vi "load_automatic.vi"(8 "error in (no error)":errorcluster) -> (0 "error out":errorcluster, 2 "replaced_step(s)":bool, 3 "automatic_steps out":variant)   [LabVIEW 2015, in "example_02.lvlib"]
doc: "load_automatic.vi will add automatic steps as variant attributes to an empty variant."
uses:
  example_02.lvlib
  <userlib>/antonio-alexander/lv-recipe-machine/public/_controls/step.ctl
  <userlib>/antonio-alexander/lv-recipe-machine/public/_controls/vi_reference_type.ctl
  _controls/steps_actions.ctl
  <userlib>/antonio-alexander/lv-recipe-machine/public/_controls/vi_reference_automatic_step.ctl
  <userlib>/antonio-alexander/lv-recipe-machine/public/_controls/vi_reference_criteria.ctl
  <userlib>/antonio-alexander/lv-recipe-machine/public/_controls/vi_reference_launch.ctl
  <userlib>/antonio-alexander/lv-recipe-machine/public/_controls/vi_reference_manual_action.ctl
  <userlib>/antonio-alexander/lv-recipe-machine/public/_controls/vi_reference_transition.ctl
  automatic_steps/transition.vi
  automatic_steps/automatic_step_address.vi
  automatic_steps/automatic_step_city.vi
  automatic_steps/automatic_step_state.vi
  automatic_steps/automatic_step_submit.vi
  automatic_steps/automatic_step_finish.vi
  <userlib>/antonio-alexander/lv-recipe-machine/lv-recipe-machine.lvlib
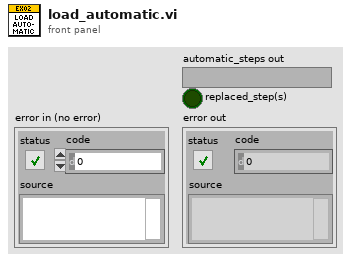
[diagram p1: front panel]
types:
  T1 = typedef "lv-recipe-machine.lvlib/vi_reference_type.ctl" = enum16{"<vi_reference_type>", "manual_action", "auto_step", "auto_criteria", "auto_transition", "auto_launcher", "<null>"}
  T2 = typedef "lv-recipe-machine.lvlib/vi_reference_transition.ctl" = refnum<vi>
  T3 = typedef "lv-recipe-machine.lvlib/vi_reference_manual_action.ctl" = refnum<vi>
  T4 = typedef "lv-recipe-machine.lvlib/vi_reference_launch.ctl" = refnum<vi>
  T5 = typedef "lv-recipe-machine.lvlib/vi_reference_criteria.ctl" = refnum<vi>
  T6 = typedef "lv-recipe-machine.lvlib/vi_reference_automatic_step.ctl" = refnum<vi>
  T7 = typedef "example_02.lvlib/steps_actions.ctl" = enum16{"<steps_actions>", "auto_start", "auto_first_name", "auto_last_name", "auto_address", "auto_city", "auto_state", "auto_zip_code", "auto_submit", "auto_finish", "transition", "<null>"}
  T8 = typedef "lv-recipe-machine.lvlib/step.ctl" = cluster{"name":string, "vi_reference":variant}
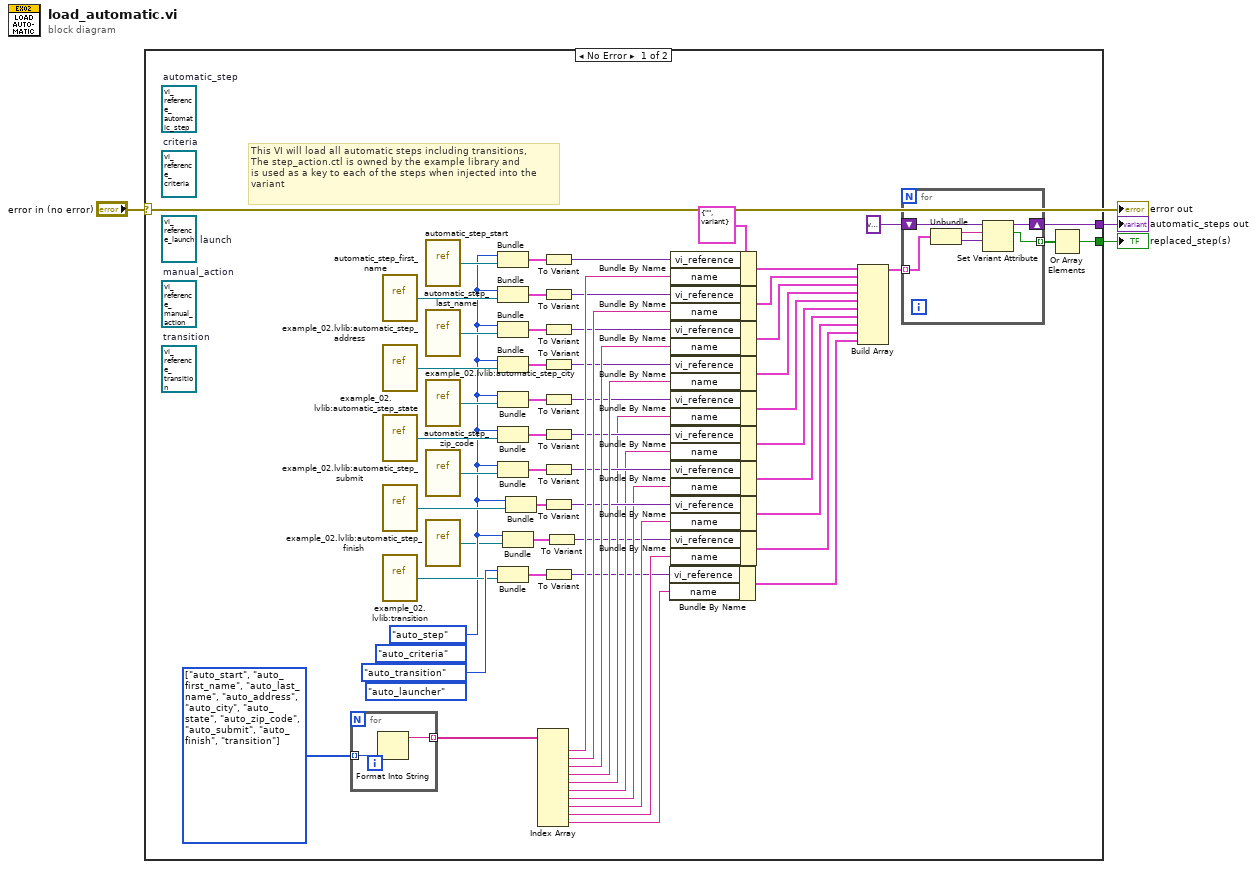
[diagram p0: block diagram]
diagram:
  n1 = case shown="No Error" "error in (no error)" {
    tunnel: [w63 _] -> w3
    tunnel: [w60 _] -> w2
    frame No Error {
      (unwired) T2 refnum  # transition
      (unwired) T3 refnum  # manual_action
      (unwired) T4 refnum  # launch
      (unwired) T5 refnum  # criteria
      (unwired) T6 refnum  # automatic_step
      (unwired) vi_reference_type."auto_launcher" ("vi_reference_type")
      w55 = T7[] [enum."auto_start", enum."auto_first_name", enum."auto_last_name", enum."auto_address", enum."auto_city", enum."auto_state", enum."auto_zip_code", enum."auto_submit", enum."auto_finish", enum."transition"] items=["<steps_actions>", "auto_start", "auto_first_name", "auto_last_name", "auto_address", "auto_city", "auto_state", "auto_zip_code", "auto_submit", "auto_finish", "transition", "<null>"]
      (unwired) vi_reference_type."auto_criteria" ("vi_reference_type")
      w8 = vi_reference_type."auto_step" ("vi_reference_type")
      w11 = T8 {"name"="", "vi_reference"=variant(refnum<vi> refnum)} ("step")
      # "This VI will load all automatic steps including transitions, \nThe step_action.ctl is owned by the example library and\nis used as a key to each of the steps when injected into the\nvariant"
      n2 = for {
        tunnel: w55 -> [w65] mode=indexing
        tunnel: [w64] -> w54 mode=indexing
        n3 = Format Into String(w65) -> (resulting string=w64:string)  [unwired: 3 in, 1 out]
      }
      n4 = vi-ref "automatic_step_first_name.vi"() -> (w48:refnum<vi>)
      n5 = vi-ref "example_02.lvlib:automatic_step_address.vi"() -> (w36:refnum<vi>)
      n6 = vi-ref "example_02.lvlib:automatic_step_state.vi"() -> (w33:refnum<vi>)
      n7 = vi-ref "example_02.lvlib:automatic_step_submit.vi"() -> (w16:refnum<vi>)
      n8 = vi-ref "example_02.lvlib:transition.vi"() -> (w38:refnum<vi>)
      n9 = vi-ref "automatic_step_start.vi"() -> (w52:refnum<vi>)
      n10 = vi-ref "automatic_step_last_name.vi"() -> (w39:refnum<vi>)
      n11 = vi-ref "example_02.lvlib:automatic_step_city.vi"() -> (w34:refnum<vi>)
      n12 = vi-ref "automatic_step_zip_code.vi"() -> (w32:refnum<vi>)
      n13 = vi-ref "example_02.lvlib:automatic_step_finish.vi"() -> (w7:refnum<vi>)
      n14 = Bundle("vi_reference_type"=w8, w52) -> (w57:cluster{"vi_reference_type":T1, refnum<vi>})  [unwired: 1 in]
      n15 = Bundle("vi_reference_type"=w8, w48) -> (w51:cluster{"vi_reference_type":T1, refnum<vi>})  [unwired: 1 in]
      n16 = Bundle("vi_reference_type"=w8, w39) -> (w37:cluster{"vi_reference_type":T1, refnum<vi>})  [unwired: 1 in]
      n17 = Bundle("vi_reference_type"=w8, w36) -> (w35:cluster{"vi_reference_type":T1, refnum<vi>})  [unwired: 1 in]
      n18 = Bundle("vi_reference_type"=w8, w34) -> (w31:cluster{"vi_reference_type":T1, refnum<vi>})  [unwired: 1 in]
      n19 = Bundle("vi_reference_type"=w8, w33) -> (w30:cluster{"vi_reference_type":T1, refnum<vi>})  [unwired: 1 in]
      n20 = Bundle("vi_reference_type"=w8, w32) -> (w29:cluster{"vi_reference_type":T1, refnum<vi>})  [unwired: 1 in]
      n21 = Bundle("vi_reference_type"=vi_reference_type."auto_transition", w38) -> (w12:cluster{"vi_reference_type":T1, refnum<vi>})  [unwired: 1 in]
      n22 = Bundle("vi_reference_type"=w8, w7) -> (w6:cluster{"vi_reference_type":T1, refnum<vi>})  [unwired: 1 in]
      n23 = Bundle("vi_reference_type"=w8, w16) -> (w15:cluster{"vi_reference_type":T1, refnum<vi>})  [unwired: 1 in]
      n24 = Index Array(array=w54) -> (element #1=w53:string, element #2=w47:string, element #3=w46:string, element #4=w41:string, element #5=w24:string, element #6=w23:string, element #7=w22:string, element #8=w21:string, element #9=w13:string, element #10=w4:string)  [unwired: 10 in]
      n25 = To Variant(anything=w57) -> (Variant=w58:variant)
      n26 = To Variant(anything=w51) -> (Variant=w49:variant)
      n27 = To Variant(anything=w37) -> (Variant=w45:variant)
      n28 = To Variant(anything=w35) -> (Variant=w40:variant)
      n29 = To Variant(anything=w31) -> (Variant=w28:variant)
      n30 = To Variant(anything=w30) -> (Variant=w27:variant)
      n31 = To Variant(anything=w29) -> (Variant=w26:variant)
      n32 = To Variant(anything=w15) -> (Variant=w25:variant)
      n33 = To Variant(anything=w12) -> (Variant=w9:variant)
      n34 = To Variant(anything=w6) -> (Variant=w5:variant)
      n35 = Bundle By Name(cluster=w11, "vi_reference"=w9, "name"=w4) -> (w10:T8)
      n36 = Bundle By Name(cluster=w11, "vi_reference"=w58, "name"=w53) -> (w56:T8)
      n37 = Bundle By Name(cluster=w11, "vi_reference"=w49, "name"=w47) -> (w50:T8)
      n38 = Bundle By Name(cluster=w11, "vi_reference"=w45, "name"=w46) -> (w44:T8)
      n39 = Bundle By Name(cluster=w11, "vi_reference"=w40, "name"=w41) -> (w42:T8)
      n40 = Bundle By Name(cluster=w11, "vi_reference"=w28, "name"=w24) -> (w20:T8)
      n41 = Bundle By Name(cluster=w11, "vi_reference"=w27, "name"=w23) -> (w19:T8)
      n42 = Bundle By Name(cluster=w11, "vi_reference"=w26, "name"=w22) -> (w18:T8)
      n43 = Bundle By Name(cluster=w11, "vi_reference"=w25, "name"=w21) -> (w17:T8)
      n44 = Bundle By Name(cluster=w11, "vi_reference"=w5, "name"=w13) -> (w14:T8)
      n45 = Build Array(w56, w50, w44, w42, w20, w19, w18, w17, w14, w10) -> (w62:T8[])
      n46 = for {
        tunnel: w62 -> [w69] mode=indexing
        shift-right: [w70] -> w63
        shift-left: variant ("automatic_steps in") -> [w71]
        tunnel: [w67] -> w59 mode=indexing
        n47 = Unbundle(w69) -> ("name"=w68:string, "vi_reference"=w66:variant)
        n48 = Set Variant Attribute(Variant=w71, name=w68, value=w66) -> (Variant out=w70:variant, replaced=w67:bool)  [unwired: 1 in, 1 out]
      }
      n49 = Or Array Elements(Boolean array=w59) -> (logical OR=w60:bool)
    }
    frame Error {
    }
  }
  "automatic_steps out" <- w3
  "replaced_step(s)" <- w2
  "error out" <- "error in (no error)"
